vi "GetControlVariantValueOrNull.vi"(11 "ControlVariant":variant) -> (0 "IsControl":bool, 3 "Value":variant)   [LabVIEW 2017]
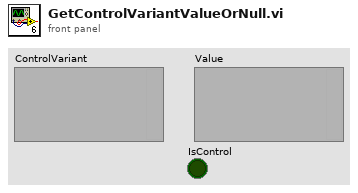
[diagram p1: front panel]
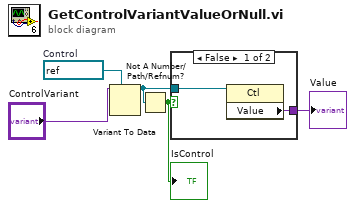
[diagram p0: block diagram]
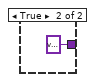
[diagram p2: hidden frame]
diagram:
  w2 = refnum<vi> refnum  # Control
  n1 = Variant To Data(type=w2, Variant="ControlVariant") -> (data=w4:refnum<vi>)  [unwired: 1 in, 1 out]
  n2 = Not A Number/Path/Refnum?(number/path/refnum=w4) -> (NaN/Path/Refnum?=w3:bool)
  "IsControl" <- w3
  n3 = case shown="False" w3 {
    tunnel: w4 -> [w7 _]
    tunnel: [w6 variant ("Value")] -> w5
    frame False {
      n4 = property class="Ctl"(reference=w7) -> ("Value"=w6:variant)  [unwired: 1 in, 2 out]
    }
    frame True {
    }
  }
  "Value" <- w5
